vi "Uncompress Becker-Hickl Data.vi"(8 "error in (no error)":errorcluster, 11 "Compressed Data in":u8[](array[numeric])) -> (0 "error out":errorcluster, 1 "size in":i32, 2 "size out":i32, 3 "Uncompressed Data out":u8[](array[numeric]))   [LabVIEW 2021, in "Becker-Hickl Files.lvlib"]
uses:
  Becker-Hickl Files.lvlib
  <vilib>/zip/NI_Unzip.lvlib
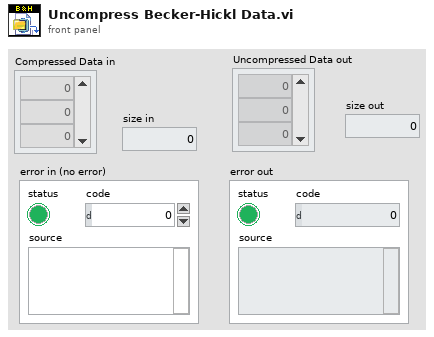
[diagram p1: front panel]
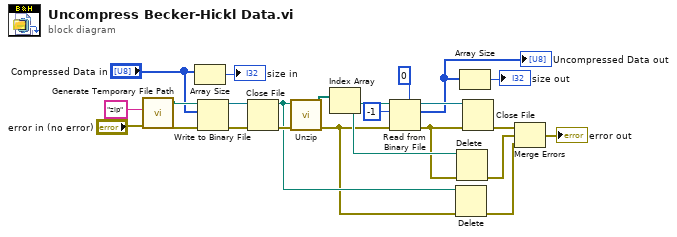
[diagram p0: block diagram]
diagram:
  n1 = call <vilib>:"Generate Temporary File Path.vi"("error in (no error)"="error in (no error)", "Temporary File Extension (tmp)"="zip") -> ("error out"=w16:errorcluster, "Unique Temporary File Path"=w15:path)  [unwired: 8 in]
  n2 = Array Size(array="Compressed Data in") -> (size(s)=→"size in":i32)
  n3 = Write to Binary File(file (use dialog)=w15, data="Compressed Data in", error in=w16) -> (refnum out=w13:refnum<file>, error out=w23:errorcluster)  [unwired: 3 in, 1 out]
  n4 = Close File(refnum=w13, error in=w23) -> (path=w11:path, error out=w14:errorcluster)
  n5 = call <vilib>:"Unzip.vi"("error in (no error)"=w14, "Zip file"=w11) -> ("error out"=w8:errorcluster, "Unzipped files"=w22:path[])  [unwired: 7 in, 1 out]
  n6 = Index Array(array=w22) -> (element=w10:path)  [unwired: 1 in]
  n7 = Read from Binary File(5:u8 0 ("count (1)"), 8:w8, 10:-1 ("count (1)"), 11:w10) -> (0:w9:errorcluster, 2:w1:u8[], 3:w18:refnum<file>)  [unwired: 2 in, 1 out]
  "Uncompressed Data out" <- w1
  n8 = Delete(path (use dialog)=w11, error in=w8) -> (error out=w5:errorcluster)  [unwired: 3 in, 2 out]
  n9 = Delete(path (use dialog)=w10, error in=w9) -> (error out=w6:errorcluster)  [unwired: 3 in, 2 out]
  n10 = Array Size(array=w1) -> (size(s)=→"size out":i32)
  n11 = Close File(refnum=w18, error in=w9) -> (error out=w19:errorcluster)  [unwired: 1 out]
  n12 = Merge Errors(w19, w6, w5) -> (→"error out":errorcluster)
